vi "scaraforward.vi"(8 "L2":dbl=1.0 format="%#_13g", 9 "L1":dbl=1.0 format="%#_13g", 10 "Angle2":dbl, 11 "Angle1":dbl) -> (2 "Y":dbl=1.0 format="%#_13g", 3 "X":dbl=1.0 format="%#_13g")   [LabVIEW 2017]
panel:
  in  "Y0":dbl=1.0 format="%#_13g"
  in  "X0":dbl format="%#_13g"
  in  "L3":dbl=1.0 format="%#_13g"
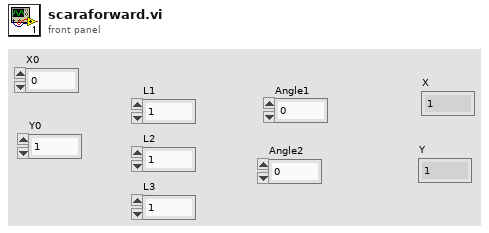
[diagram p1: front panel]
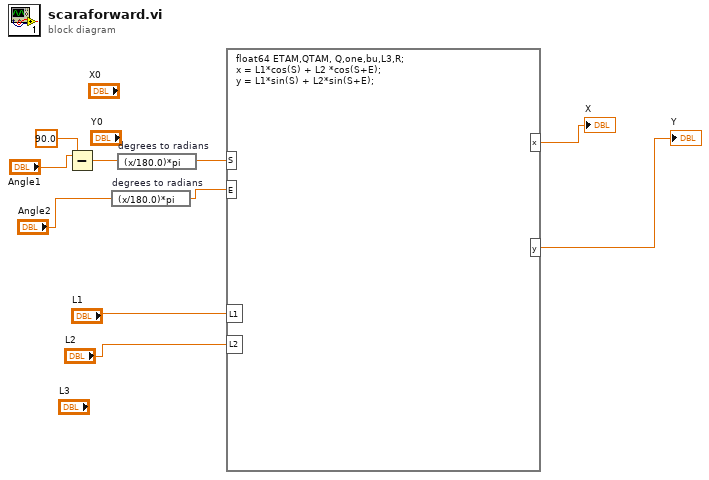
[diagram p0: block diagram]
diagram:
  n1 = Subtract(x="Angle1", y=90.0) -> (x-y=w3:dbl)
  n2 = expression code="(x/180.0)*pi" "degrees to radians"("Angle2") -> (w6:dbl)
  n3 = expression code="(x/180.0)*pi" "degrees to radians"(w3) -> (w7:dbl)
  n4 = formula code="float64 ETAM,QTAM, Q,one,bu,L3,R;\nx = L1*cos(S) + L2 *cos(S+E);\ny = L1*sin(S) + L2*sin(S+E);"("S"=w7, "E"=w6, "L1"="L1", "L2"="L2") -> ("x"=→"X":dbl, "y"=→"Y":dbl)
